vi "Setup subWorker - Status Platine Newport.vi"(8 "error in":errorcluster, 11 "UI SmarAct in":refnum<class "UI SmarAct.lvclass">) -> (0 "error out":errorcluster, 3 "UI SmarAct out":refnum<class "UI SmarAct.lvclass">)   [LabVIEW 2024, in "UI SmarAct.lvclass"]
doc: "This VI sets up the framework parameters of a statically-linked subWorker."
uses:
  UI SmarAct.lvclass
  UI SmarAct.lvclass/UI SmarAct.ctl
  Status Platine Newport/Status Platine Newport.lvclass
  C:/Program Files (x86)/National Instruments/LabVIEW 2024/vi.lib/addons/_Workers/Library/Classes/Worker/Worker.lvclass
  C:/Program Files (x86)/National Instruments/LabVIEW 2024/vi.lib/addons/_Workers/Library/Classes/Workers Object/Workers Object.lvclass
  C:/Users/flepetit/Desktop/FROG-SHG-LV2024/Workers/Status Platine Newport/Status Platine Newport.lvclass
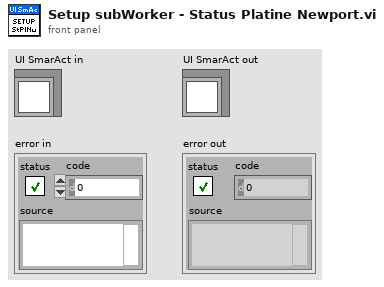
[diagram p1: front panel]
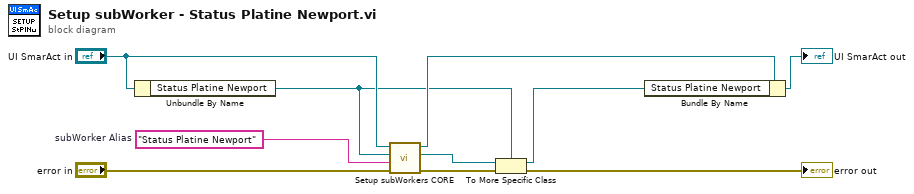
[diagram p0: block diagram]
diagram:
  w6 = "Status Platine Newport"  # subWorker Alias
  n1 = Unbundle By Name("UI SmarAct in") -> ("Status Platine Newport"=w3:refnum<class "Status Platine Newport.lvclass">)
  n2 = call-dynamic "Setup subWorkers CORE.vi"("error in"="error in", "subWorker Alias"=w6, "subWorker"=w3, "Worker"="UI SmarAct in") -> ("error out"=w5:errorcluster, "subWorker out"=w1:refnum<class "Worker.lvclass">, "Worker out"=w8:refnum<class "UI SmarAct.lvclass">)  [unwired: 5 in]
  n3 = To More Specific Class(target class=w3, reference=w1, error in=w5) -> (specific class reference=w2:refnum<class "Status Platine Newport.lvclass">, error out=→"error out":errorcluster)
  n4 = Bundle By Name(cluster=w8, "Status Platine Newport"=w2) -> (→"UI SmarAct out":refnum<class "UI SmarAct.lvclass">)
